vi "Cast_String_To_Visa.vi"(11 "Inovance_Camera in":refnum<class "Inovance_Camera.lvclass">) -> (3 "Inovance Address":T1)   [LabVIEW 2023, in "Inovance_Camera.lvlib" / "Inovance_Camera.lvclass"]
uses:
  Inovance_Camera.lvclass
  <vilib>/userDefined/High Color/IMAQdx.ctl
  Inovance_Camera.lvclass/Inovance_Camera.ctl
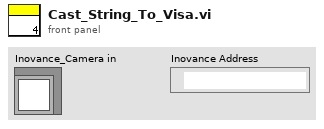
[diagram p1: front panel]
types:
  T1 = typedef "IMAQdx.ctl" = refnum<k21>
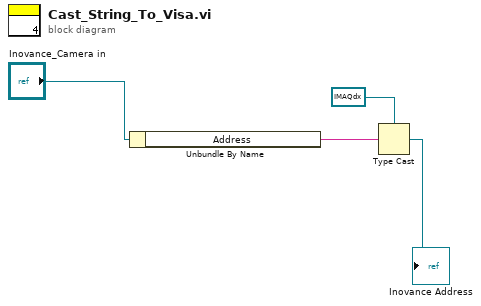
[diagram p0: block diagram]
diagram:
  n1 = Unbundle By Name("Inovance_Camera in") -> ("Address"=w3:string)
  n2 = Type Cast(type=T1 refnum ("Inovance Address"), x=w3) -> (*(type *) &x=→"Inovance Address":T1)
